vi "WS102x_Multi DUT_Calculate VCMIN.vi"(7 "Pos_Voltage(V)":dbl, 8 "error in (no error)":errorcluster, 9 "V3_VCmin":string[][](table), 10 "V2_VCmin":string[][](table), 11 "V1_VCmin":string[][](table)) -> (0 "error out":errorcluster, 3 "VCmin":string[][](array[string]))   [LabVIEW 2017]
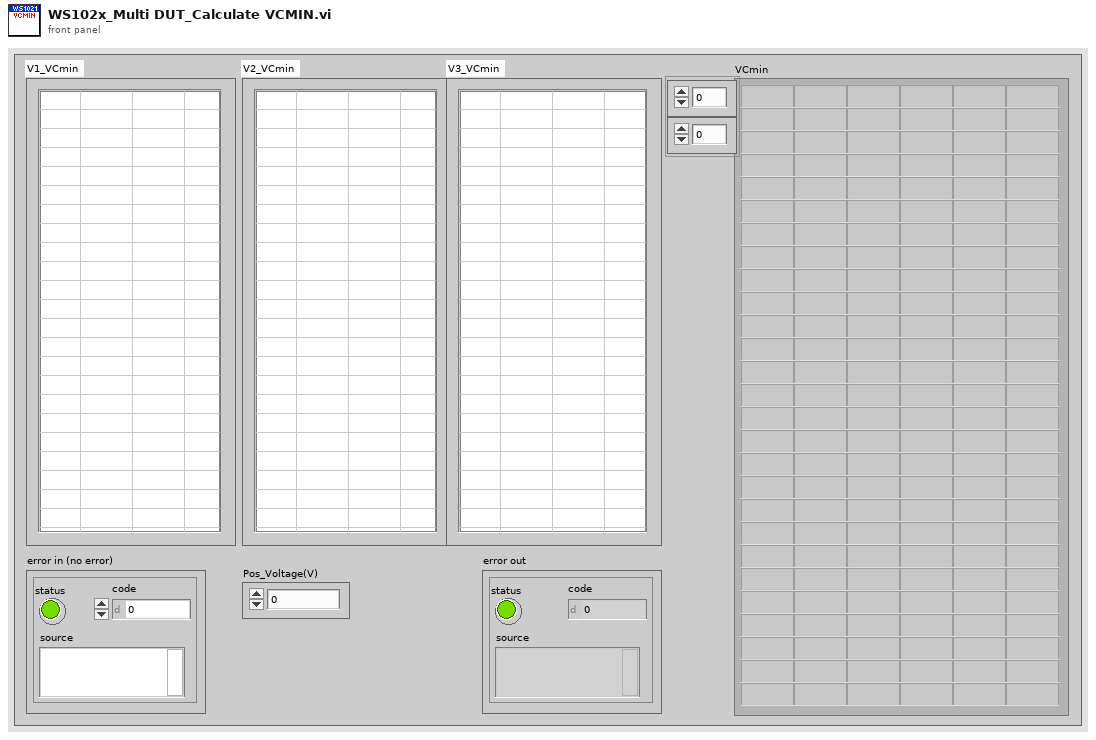
[diagram p1: front panel]
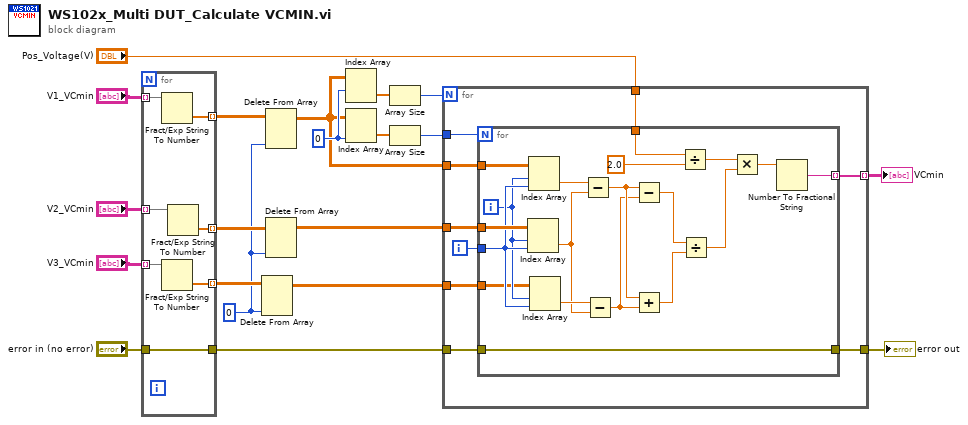
[diagram p0: block diagram]
diagram:
  w1 = 0 ("disabled index (col)")
  w13 = 0 ("index (row)")
  n1 = for {
    tunnel: "V1_VCmin" -> [w27] mode=indexing
    tunnel: "V2_VCmin" -> [w26] mode=indexing
    tunnel: "V3_VCmin" -> [w25] mode=indexing
    tunnel: [w24] -> w7 mode=indexing
    tunnel: [w23] -> w5 mode=indexing
    tunnel: [w22] -> w3 mode=indexing
    tunnel: "error in (no error)" -> [w21]
    tunnel: [w21] -> w9
    n2 = Fract/Exp String To Number(string=w27) -> (number=w24:dbl[])  [unwired: 3 in, 1 out]
    n3 = Fract/Exp String To Number(string=w25) -> (number=w22:dbl[])  [unwired: 3 in, 1 out]
    n4 = Fract/Exp String To Number(string=w26) -> (number=w23:dbl[])  [unwired: 3 in, 1 out]
  }
  n5 = Delete From Array(array=w3, index (col)=w1) -> (array with subset deleted=w2:dbl[][])  [unwired: 2 in, 1 out]
  n6 = Delete From Array(array=w7, index (col)=w1) -> (array with subset deleted=w6:dbl[][])  [unwired: 2 in, 1 out]
  n7 = Delete From Array(array=w5, index (col)=w1) -> (array with subset deleted=w4:dbl[][])  [unwired: 2 in, 1 out]
  n8 = Index Array(array=w6, index (row)=w13) -> (element=w14:dbl[])  [unwired: 1 in]
  n9 = Index Array(array=w6, index (col)=w13) -> (element=w16:dbl[])  [unwired: 1 in]
  n10 = Array Size(array=w14) -> (size(s)=w15:i32)
  n11 = Array Size(array=w16) -> (size(s)=w17:i32)
  n12 = for {
    N: w15 -> [_]
    tunnel: w17 -> [w36]
    tunnel: w6 -> [w35]
    tunnel: w4 -> [w34]
    tunnel: w2 -> [w32]
    tunnel: "Pos_Voltage(V)" -> [w31]
    tunnel: [w30] -> w11 mode=indexing
    tunnel: w9 -> [w29]
    tunnel: [w28] -> w8
    i -> [w33]
    n13 = for {
      N: w36 -> [_]
      tunnel: w35 -> [w55]
      tunnel: w34 -> [w54]
      tunnel: w33 -> [w52]
      tunnel: w32 -> [w50]
      tunnel: w31 -> [w45]
      tunnel: [w40] -> w30 mode=indexing
      tunnel: w29 -> [w39]
      tunnel: [w39] -> w28
      i -> [w51]
      n14 = Index Array(array=w54, index (row)=w51, index (col)=w52) -> (element=w48:dbl)
      n15 = Index Array(array=w55, index (row)=w51, index (col)=w52) -> (element=w53:dbl)
      n16 = Index Array(array=w50, index (row)=w51, index (col)=w52) -> (element=w49:dbl)
      n17 = Subtract(x=w53, y=w48) -> (x-y=w38:dbl)
      n18 = Subtract(x=w49, y=w48) -> (x-y=w37:dbl)
      n19 = Subtract(x=w38, y=w37) -> (x-y=w47:dbl)
      n20 = Add(x=w38, y=w37) -> (x+y=w46:dbl)
      n21 = Divide(x=w45, y=2.0) -> (x/y=w42:dbl)
      n22 = Divide(x=w47, y=w46) -> (x/y=w43:dbl)
      n23 = Multiply(x=w42, y=w43) -> (x*y=w41:dbl)
      n24 = Number To Fractional String(number=w41) -> (F-format string=w40:string)  [unwired: 3 in]
    }
  }
  "VCmin" <- w11
  "error out" <- w8
